vi "Cleanup.vi"(8 "error in (no error)":errorcluster, 11 "Effect Interface in":refnum<class "Effect Interface.lvclass">) -> (0 "error out":errorcluster, 3 "Effect Interface out":refnum<class "Effect Interface.lvclass">)   [LabVIEW 2019, in "Effect Interface.lvlib" / "Effect Interface.lvclass"]
uses:
  Effect Interface.lvclass
  Effect Interface.lvclass/Effect Interface.ctl
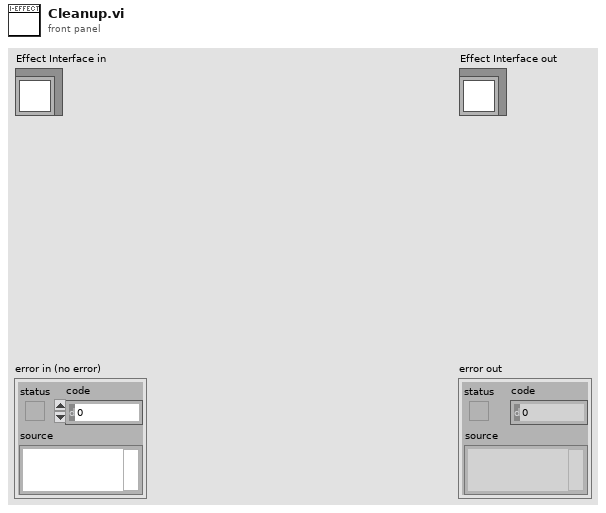
[diagram p1: front panel]
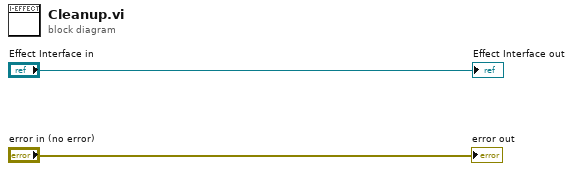
[diagram p0: block diagram]
diagram:
  "error out" <- "error in (no error)"
  "Effect Interface out" <- "Effect Interface in"
